vi "Stop.vi"(8 "error in (no error)":errorcluster, 11 "Application in":refnum<data-value>) -> (0 "error out":errorcluster, 3 "Application out":refnum<data-value>)   [LabVIEW 2015, in "Application.lvclass"]
uses:
  Application.lvclass
  Project.lvclass
  Plugin.lvclass
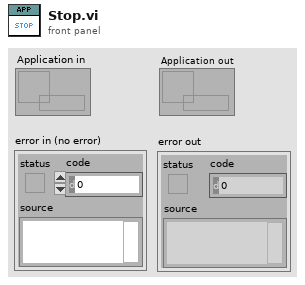
[diagram p1: front panel]
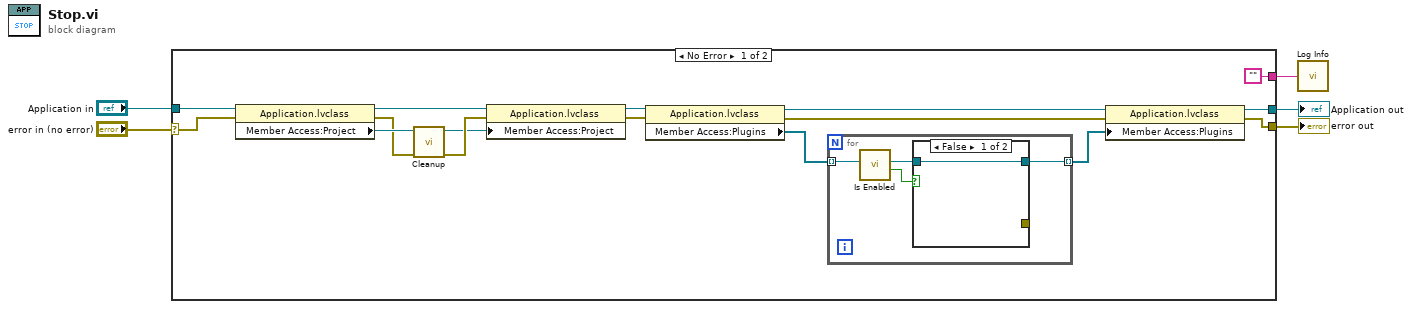
[diagram p0: block diagram]
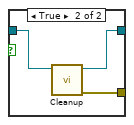
[diagram p2: hidden frame]
diagram:
  n1 = case shown="No Error" "error in (no error)" {
    selector: "error in (no error)" -> [w15 w31]
    tunnel: [w8 w31] -> w4
    tunnel: [w10 w30] -> w1
    tunnel: "Application in" -> [w21 w30]
    tunnel: ["" _] -> w3
    frame No Error {
      n2 = property class="Application.lvclass"(reference=w21, error in=w15) -> (reference out=w18:refnum<data-value>, error out=w19:errorcluster, "Member Access:Project"=w20:refnum<class "Project.lvclass">)
      n3 = call-dynamic "Cleanup.vi"("error in (no error)"=w19, "ProjectBase in"=w20) -> ("error out"=w17:errorcluster, "ProjectBase out"=w16:refnum<class "Project.lvclass">)  [unwired: 8 in]
      n4 = property class="Application.lvclass"(reference=w18, error in=w17, "Member Access:Project"=w16) -> (reference out=w13:refnum<data-value>, error out=w12:errorcluster)
      n5 = property class="Application.lvclass"(reference=w13, error in=w12) -> (reference out=w9:refnum<data-value>, error out=w6:errorcluster, "Member Access:Plugins"=w11:refnum<class "Plugin.lvclass">[])
      n6 = for {
        tunnel: w11 -> [w24] mode=indexing
        tunnel: [w25] -> w7 mode=indexing
        n7 = call "Is Enabled.vi"("Plugin in"=w24) -> ("Enabled"=w22:bool, "Plugin out"=w23:refnum<class "Plugin.lvclass">)  [unwired: 9 in]
        n8 = case shown="False" w22 {
          tunnel: [_ w29] -> _
          tunnel: [w26 w28] -> w25
          tunnel: w23 -> [w26 w27]
          frame False {
          }
          frame True {
            n9 = call-dynamic "Cleanup.vi"("Plugin in"=w27) -> ("error out"=w29:errorcluster, "Plugin out"=w28:refnum<class "Plugin.lvclass">)  [unwired: 9 in]
          }
        }
      }
      n10 = property class="Application.lvclass"(reference=w9, error in=w6, "Member Access:Plugins"=w7) -> (reference out=w10:refnum<data-value>, error out=w8:errorcluster)
    }
    frame Error {
    }
  }
  "error out" <- w4
  "Application out" <- w1
  n11 = call "Log Info.vi"("Message"=w3) -> ()  [unwired: 4 in, 1 out]
